vi "3D Control Practice.vi"() -> ()   [LabVIEW 2021]
uses:
  <vilib>/Utility/miscctls.llb/LV3DPointTypeDef.ctl
  <vilib>/picture/3D Picture Control/Object/Create Object (drawable).vi
  <vilib>/picture/3D Picture Control/Object/Add Object (no reference).vi
  <vilib>/picture/3D Picture Control/NI_3D Picture Control.lvlib
panel:
  in  "Axis 1 Degrees":sgl(slide) min=0 max=360 step=1 scale=0.0..360.0
  in  "Axis":T1
  in  "Wall":dbl(slide)=0.5 min=0.0 max=1.0 step=0.05 scale=0.0..1.0
  in  "Background":u32(colorbox)=5789784
  in  "Axis Color":u32(colorbox)=16448250
  in  "Wall Color":u32(colorbox)=6618880
  in  "Machine Color":u32(colorbox)=16711680
  in  "stop":bool
  out "Test Area":refnum<vi>(3d-picture)
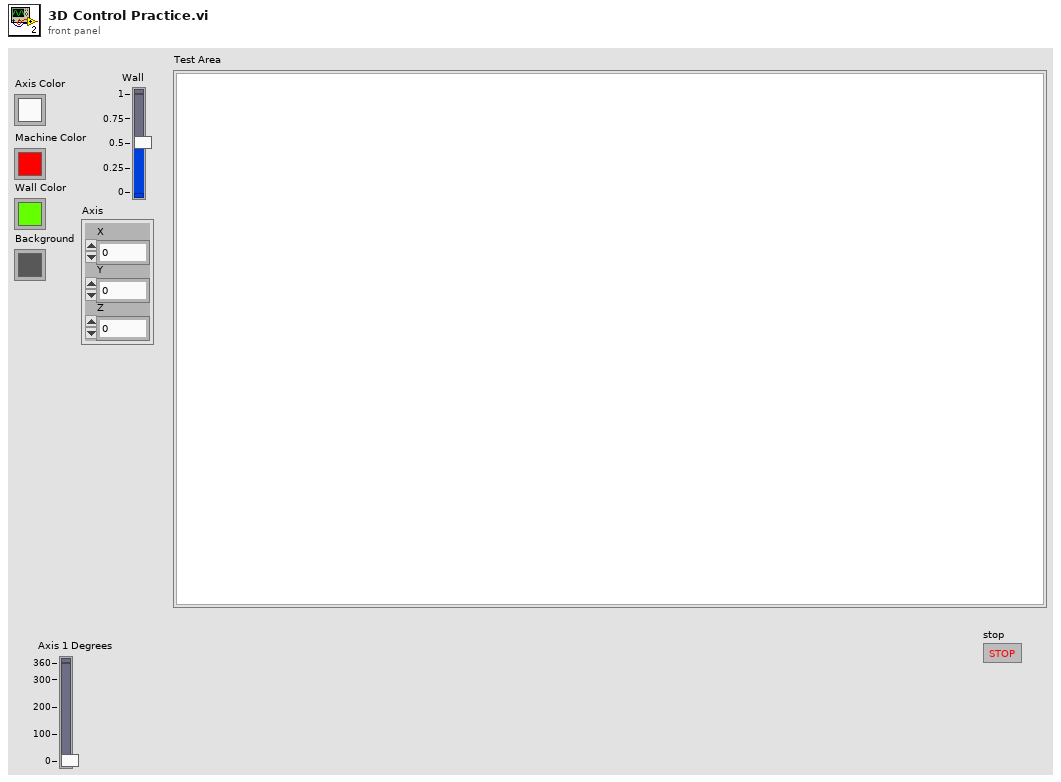
[diagram p1: front panel]
types:
  T1 = typedef "LV3DPointTypeDef.ctl" = cluster{"X":sgl, "Y":sgl, "Z":sgl}
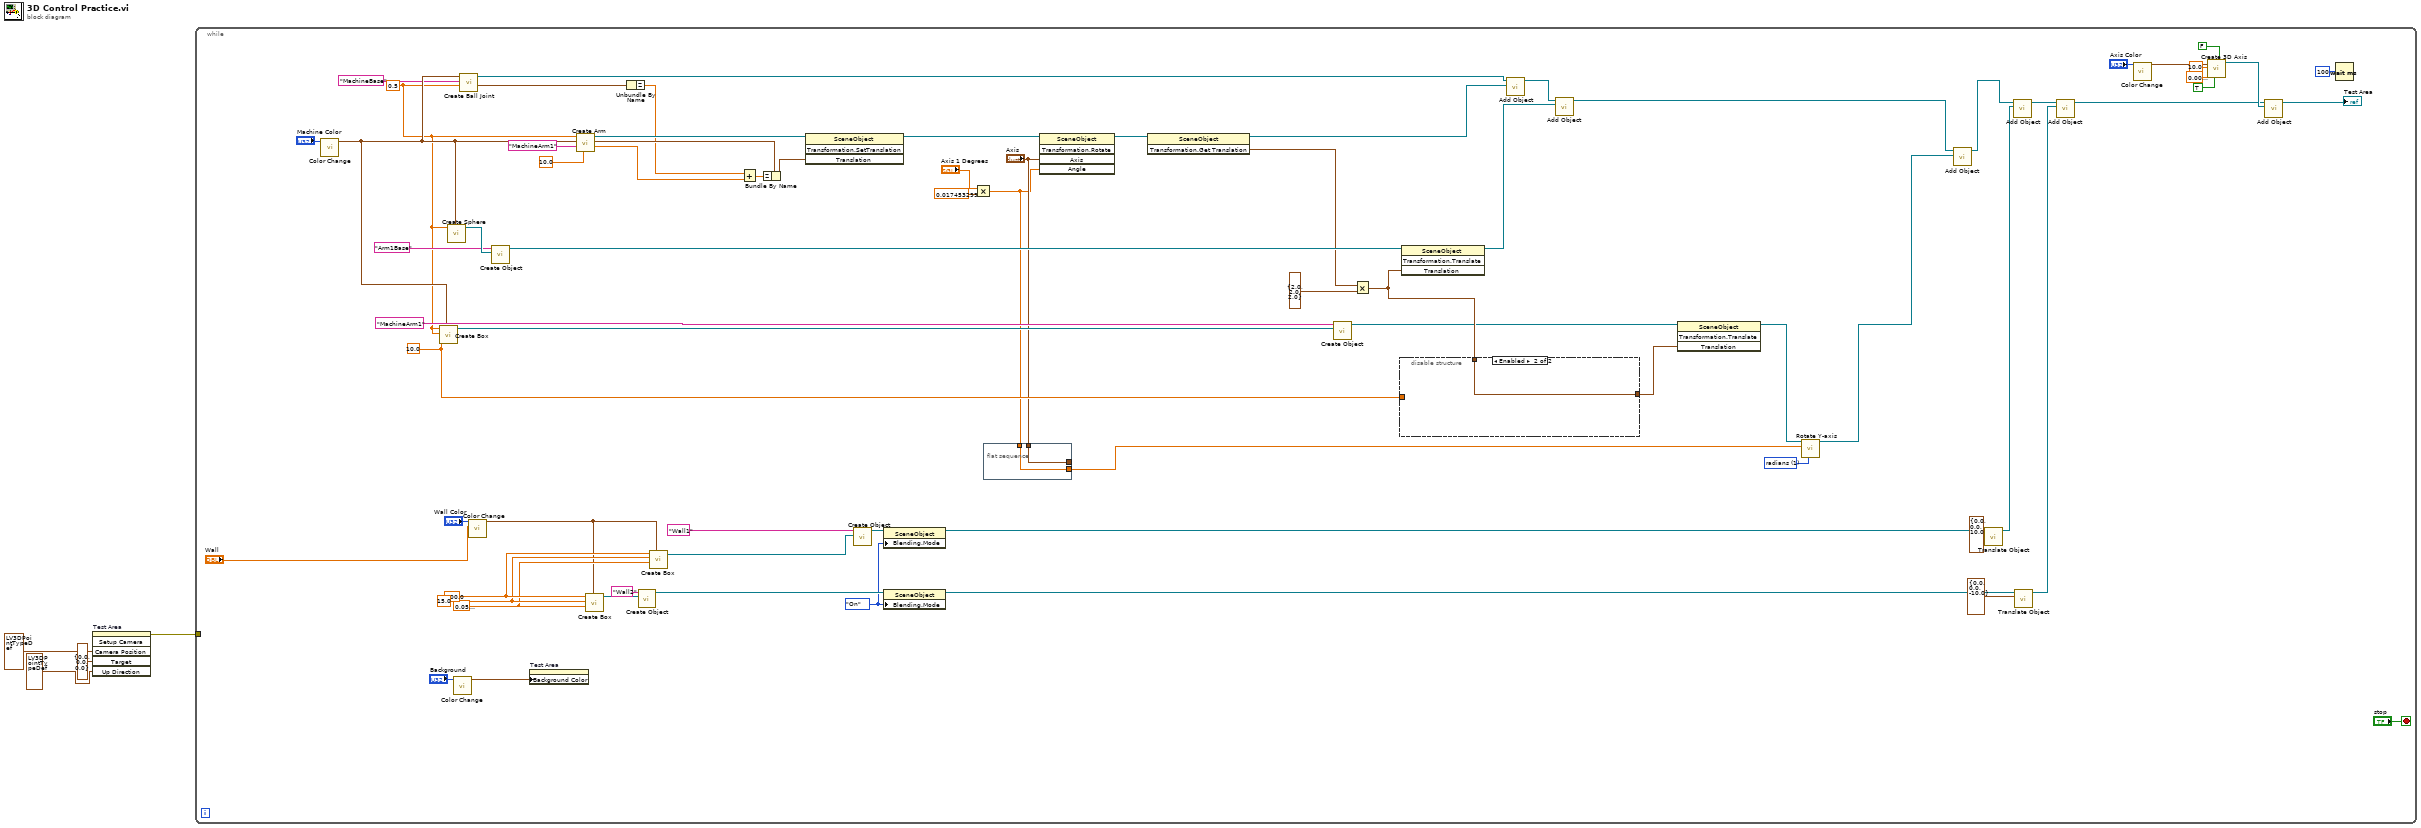
[diagram p0: block diagram]
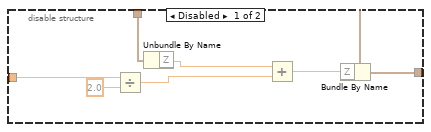
[diagram p2: hidden frame]
diagram:
  n1 = invoke on="Test Area" class="SceneGraphDisp (strict)" method="Setup Camera"("Camera Position"=T1 {"X"=25.4, "Y"=40.2, "Z"=20.3}, "Target"=T1 {"X"=0.0, "Y"=0.0, "Z"=0.0}, "Up Direction"=T1 {"X"=0.2, "Y"=0.3, "Z"=0.4}) -> (error out=w1:errorcluster)  [unwired: 3 in, 5 out]
  n2 = while {
    tunnel: w1 -> [_]
    stop <- "stop" stop-if-true
    w5 = u16 1 items=["degree", "radians"] ("angle unit")
    w16 = sgl 0.5 ("Radius 2")
    w27 = sgl 10.0 ("Length Z")
    w46 = enum16{"Inherit Value", "Off", "On"}."On" ("Blending:Mode")
    w63 = sgl 0.05 ("Length X")
    w64 = sgl 15.0 ("Length X")
    w65 = sgl 100.0 ("Length X")
    n3 = call <vilib>:"Color Change.vi"("Color"="Machine Color") -> ("RGBA"=w24:cluster{"R":sgl, "G":sgl, "B":sgl, "A":sgl})  [unwired: 10 in]
    n4 = call <vilib>:"Create Box.vi"("Color"=w24, "Length Z"=w27, "Length Y"=w16, "Length X"=w16) -> ("New Box Refnum"=w26:refnum<vi>)  [unwired: 6 in, 1 out]
    n5 = call <vilib>:"Create Sphere.vi"("Color"=w24, "Radius"=w16) -> ("New Sphere Refnum"=w33:refnum<vi>)  [unwired: 8 in, 1 out]
    n6 = call <vilib>:"Color Change.vi"("Color"="Background") -> ("RGBA"=w54:cluster{"R":sgl, "G":sgl, "B":sgl, "A":sgl})  [unwired: 10 in]
    n7 = call "Create Ball Joint.vi"("Radius 2"=w16, "Name"="MachineBase", "RGBA"=w24) -> ("Transformation.GetTranslation"=w20:T1, "SceneObject out"=w43:refnum<vi>)  [unwired: 7 in]
    n8 = call <vilib>:"Color Change.vi"("Alpha"="Wall", "Color"="Wall Color") -> ("RGBA"=w58:cluster{"R":sgl, "G":sgl, "B":sgl, "A":sgl})  [unwired: 9 in]
    n9 = call-poly <vilib>:"Create Object.vi"("Geometry"=w33, "Name"="Arm1Base") -> ("Scene:New Object"=w23:refnum<vi>)  [unwired: 8 in, 1 out]
    n10 = property on="Test Area" class="SceneGraphDisp (strict)"("Background Color"=w54) -> ()  [unwired: 2 in, 2 out]
    n11 = call "Create Arm.vi"("Length"=sgl 10.0 ("Length Z"), "Name"="MachineArm1", "Color"=w24, "Radius"=w16) -> ("Half Length"=w37:sgl, "Transformation.GetTranslation"=w41:T1, "SceneObject out"=w42:refnum<vi>)  [unwired: 5 in]
    n12 = call <vilib>:"Create Box.vi"("Color"=w58, "Length Z"=w63, "Length Y"=w64, "Length X"=w65) -> ("New Box Refnum"=w49:refnum<vi>)  [unwired: 6 in, 1 out]
    n13 = Unbundle By Name(w20) -> ("Z"=w19:sgl)
    n14 = call-poly <vilib>:"Create Object.vi"("Geometry"=w49, "Name"="Wall2") -> ("Scene:New Object"=w48:refnum<vi>)  [unwired: 8 in, 1 out]
    n15 = call <vilib>:"Create Box.vi"("Color"=w58, "Length Z"=w63, "Length Y"=w64, "Length X"=w65) -> ("New Box Refnum"=w66:refnum<vi>)  [unwired: 6 in, 1 out]
    n16 = Add(x=w19, y=w37) -> (x+y=w39:sgl)
    n17 = Bundle By Name(cluster=w41, "Z"=w39) -> (w40:T1)
    n18 = invoke class="SceneObject" method="Transformation.SetTranslation"(reference=w42, "Translation"=w40) -> (reference out=w36:refnum<vi>)  [unwired: 2 in, 3 out]
    n19 = call-poly <vilib>:"Create Object.vi"("Geometry"=w66, "Name"="Wall1") -> ("Scene:New Object"=w51:refnum<vi>)  [unwired: 8 in, 1 out]
    n20 = property class="SceneObject"(reference=w51, "Blending.Mode"=w46) -> (reference out=w50:refnum<vi>)  [unwired: 1 in, 1 out]
    n21 = property class="SceneObject"(reference=w48, "Blending.Mode"=w46) -> (reference out=w47:refnum<vi>)  [unwired: 1 in, 1 out]
    n22 = Multiply(x="Axis 1 Degrees", y=sgl 0.0174533) -> (x*y=w13:sgl)
    n23 = flat-sequence {
      tunnel: "Axis" -> [w87]
      tunnel: w13 -> [w86]
      tunnel: [w87] -> _
      tunnel: [w86] -> w6
      frame #0 {
      }
    }
    n24 = invoke class="SceneObject" method="Transformation.Rotate"(reference=w36, "Axis"="Axis", "Angle"=w13) -> (reference out=w15:refnum<vi>)  [unwired: 2 in, 4 out]
    n25 = invoke class="SceneObject" method="Transformation.Get Translation"(reference=w15) -> (reference out=w31:refnum<vi>, "Transformation.GetTranslation"=w12:T1)  [unwired: 2 in, 1 out]
    n26 = call-poly <vilib>:"Create Object.vi"("Geometry"=w26, "Name"="MachineArm1") -> ("Scene:New Object"=w9:refnum<vi>)  [unwired: 8 in, 1 out]
    n27 = Multiply(x=w12, y=T1 {"X"=2.0, "Y"=2.0, "Z"=2.0}) -> (x*y=w11:T1)
    n28 = disable-structure shown="Enabled" {
      disable-tunnel: w27 -> [w83 _]
      disable-tunnel: w11 -> [w79 w85]
      disable-tunnel: [w78 w85] -> w10
      frame Disabled {
        n29 = Divide(x=w83, y=sgl 2.0) -> (x/y=w81:sgl)
        n30 = Unbundle By Name(w79) -> ("Z"=w80:sgl)
        n31 = Add(x=w80, y=w81) -> (x+y=w82:sgl)
        n32 = Bundle By Name(cluster=w79, "Z"=w82) -> (w78:T1)
      }
      frame Enabled {
      }
    }
    n33 = invoke class="SceneObject" method="Transformation.Translate"(reference=w23, "Translation"=w11) -> (reference out=w29:refnum<vi>)  [unwired: 2 in, 3 out]
    n34 = call-poly <vilib>:"Add Object.vi"("New Object In"=w31, "Scene Object In"=w43) -> ("Scene Object Out"=w30:refnum<vi>)  [unwired: 8 in, 1 out]
    n35 = call-poly <vilib>:"Add Object.vi"("New Object In"=w29, "Scene Object In"=w30) -> ("Scene Object Out"=w22:refnum<vi>)  [unwired: 8 in, 1 out]
    n36 = invoke class="SceneObject" method="Transformation.Translate"(reference=w9, "Translation"=w10) -> (reference out=w8:refnum<vi>)  [unwired: 2 in, 3 out]
    n37 = call <vilib>:"Rotate Y-axis.vi"("angle unit"=w5, "angle"=w6, "Scene Object In"=w8) -> ("Scene Object Out"=w7:refnum<vi>)  [unwired: 7 in, 1 out]
    n38 = call-poly <vilib>:"Add Object.vi"("New Object In"=w7, "Scene Object In"=w22) -> ("Scene Object Out"=w21:refnum<vi>)  [unwired: 8 in, 1 out]
    n39 = call <vilib>:"Translate Object.vi"("Translation"=cluster{"X":sgl, "Y":sgl, "Z":sgl} {"X"=0.0, "Y"=0.0, "Z"=10.0}, "Scene.Object In"=w50) -> ("Scene.Object Out"=w77:refnum<vi>)  [unwired: 8 in, 1 out]
    n40 = call-poly <vilib>:"Add Object.vi"("New Object In"=w77, "Scene Object In"=w21) -> ("Scene Object Out"=w76:refnum<vi>)  [unwired: 8 in, 1 out]
    n41 = call <vilib>:"Translate Object.vi"("Translation"=cluster{"X":sgl, "Y":sgl, "Z":sgl} {"X"=0.0, "Y"=0.0, "Z"=-10.0}, "Scene.Object In"=w47) -> ("Scene.Object Out"=w75:refnum<vi>)  [unwired: 8 in, 1 out]
    n42 = call-poly <vilib>:"Add Object.vi"("New Object In"=w75, "Scene Object In"=w76) -> ("Scene Object Out"=w17:refnum<vi>)  [unwired: 8 in, 1 out]
    n43 = call <vilib>:"Color Change.vi"("Color"="Axis Color") -> ("RGBA"=w56:cluster{"R":sgl, "G":sgl, "B":sgl, "A":sgl})  [unwired: 10 in]
    n44 = call <vilib>:"Create 3D Axis.vi"("Half plane?"=FALSE, "Axis label?"=TRUE, "Color"=w56, "Radius"=sgl 0.01, "Length"=sgl 10.0) -> ("New Object Refnum"=w71:refnum<vi>)  [unwired: 5 in, 1 out]
    n45 = call-poly <vilib>:"Add Object.vi"("New Object In"=w71, "Scene Object In"=w17) -> ("Scene Object Out"=→"Test Area":refnum<vi>)  [unwired: 8 in, 1 out]
    n46 = Wait (ms)(milliseconds to wait=u32 100) -> ()  [unwired: 1 out]
  }
